vi "PourButtonControl.vi"(4 "Steps":i32, 6 "Prev Duty Cycle":dbl, 7 "Pour":bool, 9 "Pour Pin":T1, 10 "New Duty Cycle":dbl, 11 "Wait Time":u32) -> (3 "Numeric":dbl)   [LabVIEW 2015]
uses:
  <vilib>/myRIO/Instrument Drivers/Onboard IO/PWM/typedefs/PWM Reference.ctl
  <vilib>/myRIO/Common/Instrument Driver Framework/Utilities/typedefs/myRIO Generic Hardware Reference.ctl
  <vilib>/myRIO/Common/Instrument Driver Framework/Utilities/typedefs/Hardware Version Enum.ctl
  <vilib>/myRIO/Common/Instrument Driver Framework/Utilities/typedefs/myRIO v1.0 Reference.ctl
  <vilib>/myRIO/Common/Instrument Driver Framework/Utilities/typedefs/Generic FPGA Reference.ctl
  <vilib>/myRIO/Common/Instrument Driver Framework/myRIO v1.0/PWM/typedefs/PWM Channels Enum.ctl
  <vilib>/myRIO/Instrument Drivers/Onboard IO/PWM/typedefs/PWM Configuration.ctl
  <vilib>/myRIO/Instrument Drivers/Onboard IO/PWM/PWM.lvlib
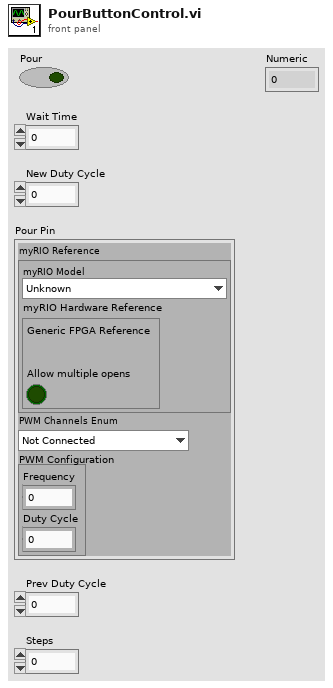
[diagram p1: front panel]
types:
  T1 = typedef "PWM.lvlib/PWM Reference.ctl" = cluster{"myRIO Reference":T2, "PWM Channels Enum":T6, "PWM Configuration":T7}
  T2 = typedef "myRIO Generic Hardware Reference.ctl" = cluster{"myRIO Model":T3, "myRIO Hardware Reference":T4}
  T3 = typedef "Hardware Version Enum.ctl" = enum16{"Unknown", "myRIO-1900", "myRIO-1950", "roboRIO"}
  T4 = typedef "myRIO v1.0 Reference.ctl" = cluster{"Generic FPGA Reference":T5, "Allow multiple opens":bool}
  T5 = typedef "Generic FPGA Reference.ctl" = refnum<k20>
  T6 = typedef "PWM Channels Enum.ctl" = enum16{"Not Connected", "C/PWM0", "C/PWM1", "A/PWM0", "A/PWM1", "A/PWM2", "B/PWM0", "B/PWM1", "B/PWM2", "PWM/PWM0", "PWM/PWM1", "PWM/PWM2", "PWM/PWM3", "PWM/PWM4", "PWM/PWM5", "PWM/PWM6", "PWM/PWM7", "PWM/PWM8", "PWM/PWM9"}
  T7 = typedef "PWM.lvlib/PWM Configuration.ctl" = cluster{"Frequency":dbl, "Duty Cycle":dbl}
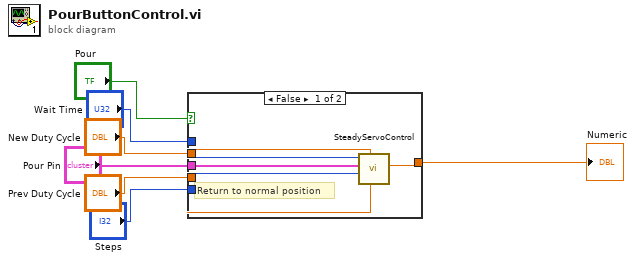
[diagram p0: block diagram]
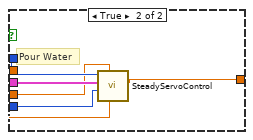
[diagram p2: hidden frame]
diagram:
  n1 = case shown="False" "Pour" {
    tunnel: "Pour Pin" -> [w13 w19]
    tunnel: "Steps" -> [w11 w18]
    tunnel: "Wait Time" -> [w12 w17]
    tunnel: "Prev Duty Cycle" -> [w10 w16]
    tunnel: "New Duty Cycle" -> [w9 w15]
    tunnel: [w8 w14] -> w7
    frame False {
      # "Return to normal position"
      n2 = call "SteadyServoControl.vi"("New Duty Cycle"=w10, "Prev Duty Cycle"=w9, "Steps"=w11, "PWM Ref Out in"=w13, "Wait Time"=w12) -> ("Numeric"=w8:dbl)  [unwired: 5 in, 1 out]
    }
    frame True {
      # "Pour Water"
      n3 = call "SteadyServoControl.vi"("New Duty Cycle"=w15, "Prev Duty Cycle"=w16, "Steps"=w18, "PWM Ref Out in"=w19, "Wait Time"=w17) -> ("Numeric"=w14:dbl)  [unwired: 5 in, 1 out]
    }
  }
  "Numeric" <- w7
